vi "child 2 define test.vi"   [LabVIEW 2013, in "Unit Tests for Runner.lvclass"]
uses:
  Unit Tests for Runner.lvclass
  classes/Test/Test.lvclass
  classes/Assert/Assert.lvclass
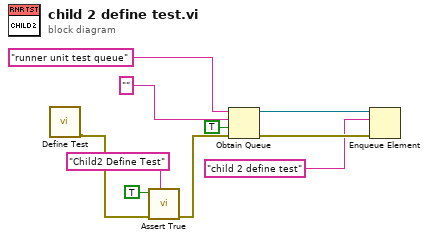
[diagram p0: block diagram]
diagram:
  n1 = call "Define Test.vi"() -> ("error out"=w2:errorcluster)  [unwired: 11 in]
  n2 = call "Assert True.vi"("Label"="Child2 Define Test", "error in (no error)"=w2, "True?"=TRUE) -> ("error out"=w1:errorcluster)  [unwired: 8 in]
  n3 = Obtain Queue(name (unnamed)="runner unit test queue", element data type="", create if not found? (T)=TRUE, error in (no error)=w1) -> (queue out=w8:refnum<queue>, error out=w7:errorcluster)  [unwired: 1 in, 1 out]
  n4 = Enqueue Element(queue=w8, element="child 2 define test", error in (no error)=w7) -> ()  [unwired: 1 in, 3 out]
